vi "Update Display Message.vi"(8 "error in (no error)":errorcluster, 10 "Wash Steps Selected-Update Display Message In":T1, 11 "Data Cluster":T2) -> (0 "error out":errorcluster, 1 "Step in progress timer control":variant, 2 "Wash Steps Selected-Update Display Message Out":T1)   [LabVIEW 2020]
doc: "Updates the Front Panel."
uses:
  Controls/Car Wash References.ctl
  Controls/Wash Steps Selected-Update Display Message.ctl
  Controls/Timer Controls.ctl
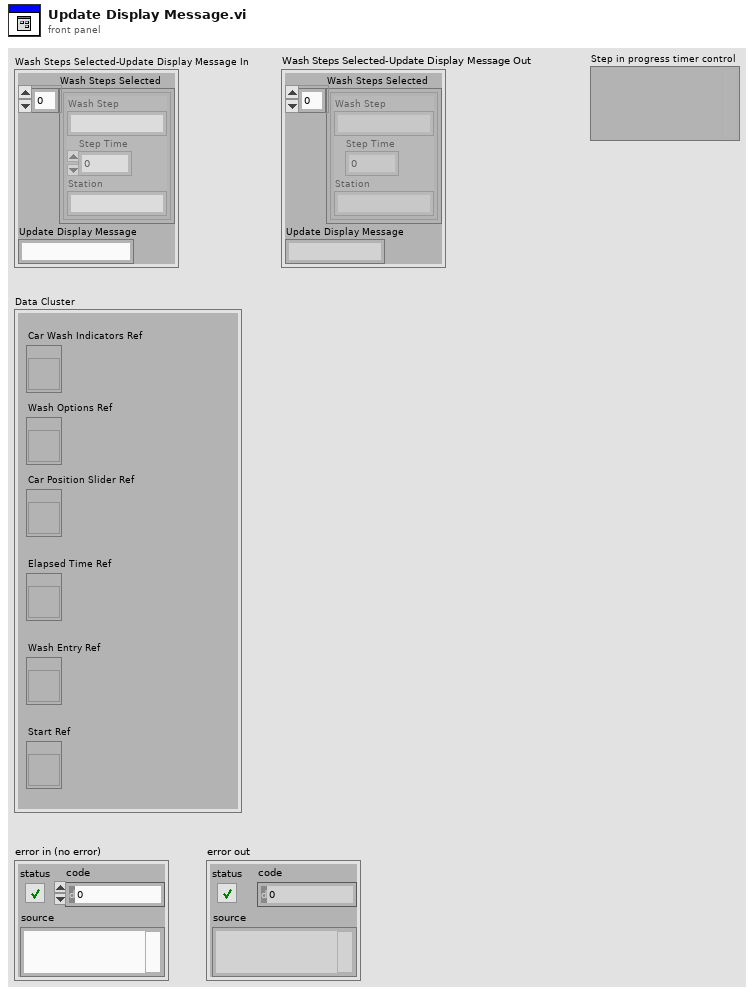
[diagram p1: front panel]
types:
  T1 = typedef "Wash Steps Selected-Update Display Message.ctl" = cluster{"Wash Steps Selected":cluster{"Wash Step":string, "Step Time":i32, "Station":string}[], "Update Display Message":string}
  T2 = typedef "Car Wash References.ctl" = cluster{"Car Wash Indicators Ref":refnum<vi>, "Wash Options Ref":refnum<vi>, "Car Position Slider Ref":refnum<vi>, "Elapsed Time Ref":refnum<vi>, "Wash Entry Ref":refnum<vi>, "Start Ref":refnum<vi>}
  T3 = enum8{"Enabled", "Disabled", "Disabled and Grayed Out"}
  T4 = cluster{"Wash Step":string, "Step Time":i32, "Station":string}[]
  T5 = typedef "Timer Controls.ctl" = enum16{"Reset", "Start", "Stop"}
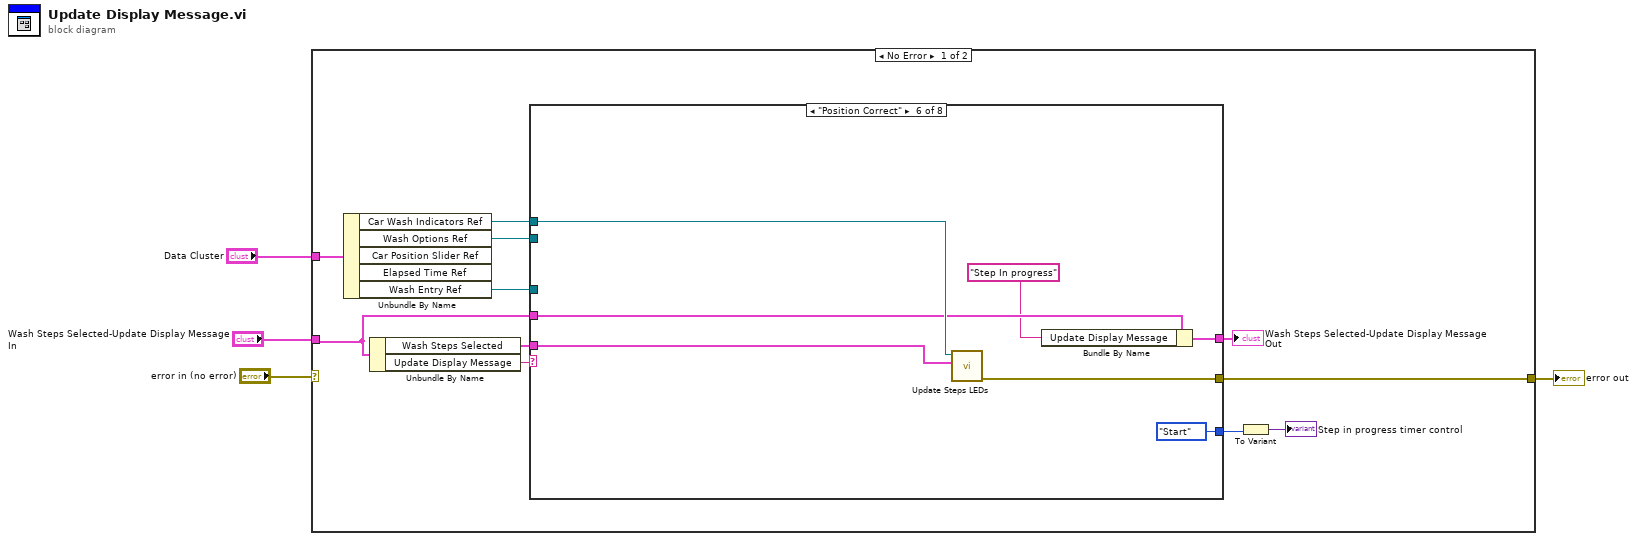
[diagram p0: block diagram]
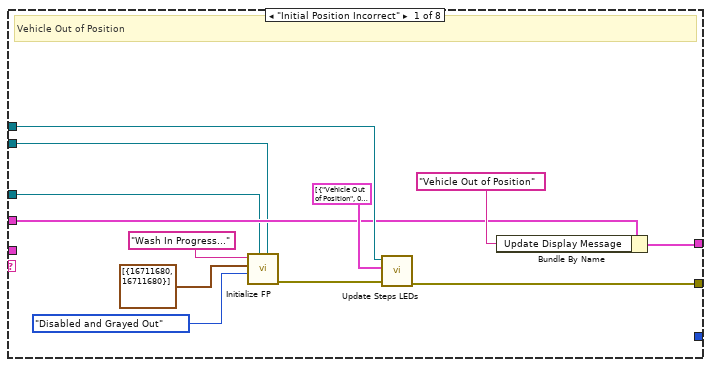
[diagram p2: hidden frame]
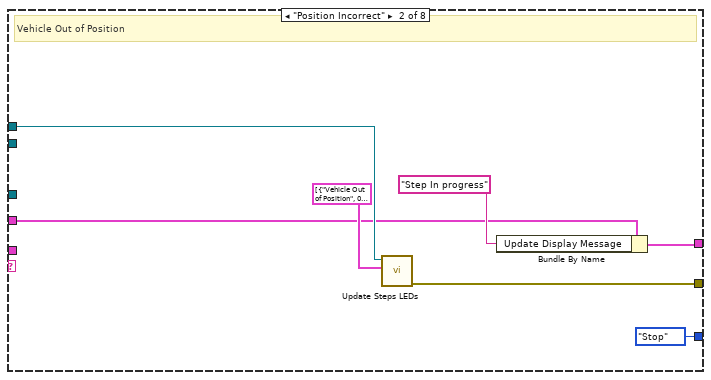
[diagram p3: hidden frame]
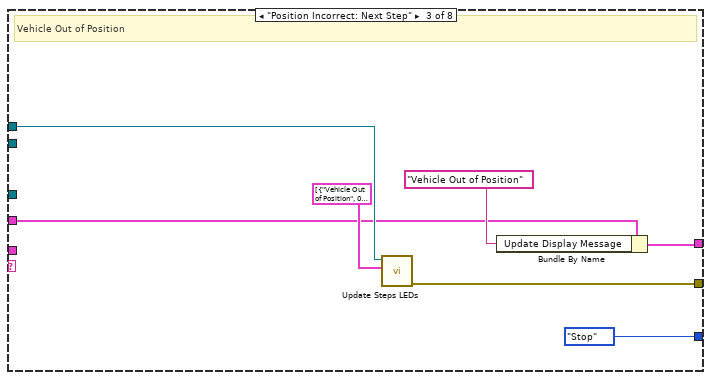
[diagram p4: hidden frame]
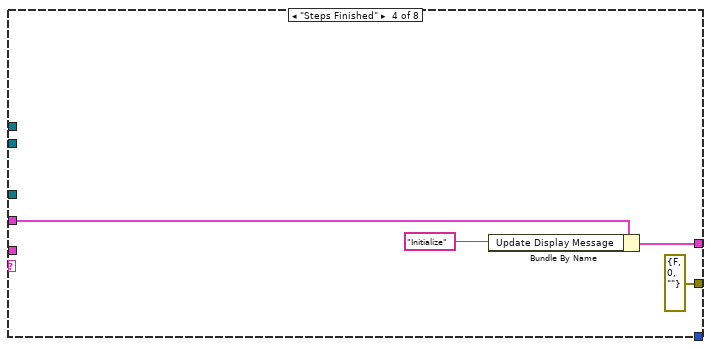
[diagram p5: hidden frame]
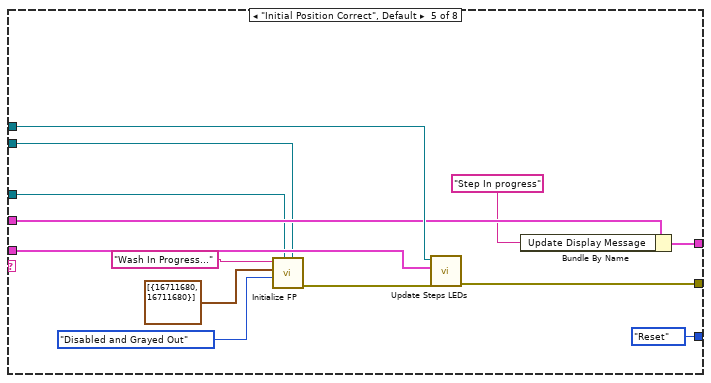
[diagram p6: hidden frame]
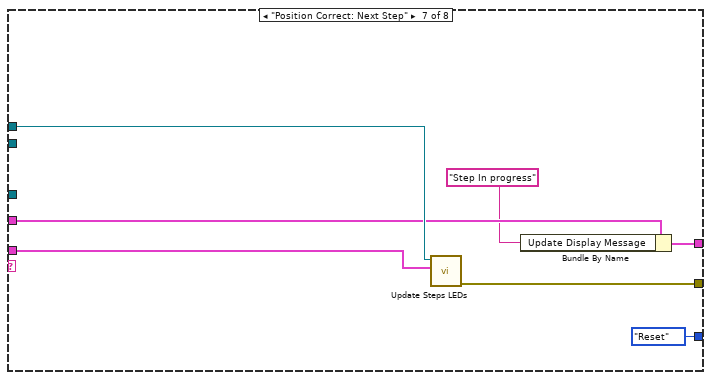
[diagram p7: hidden frame]
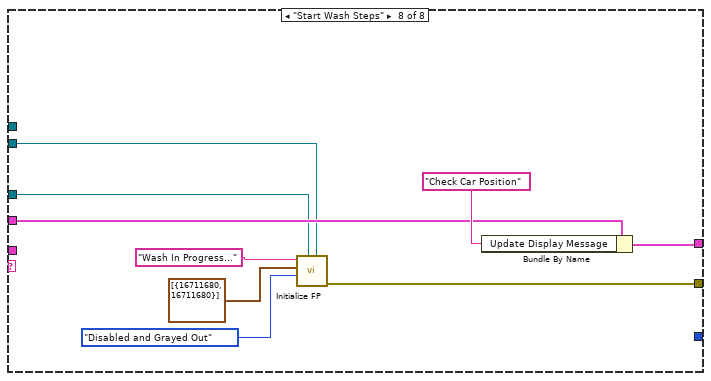
[diagram p8: hidden frame]
diagram:
  n1 = case shown="No Error" "error in (no error)" {
    selector: "error in (no error)" -> [_ w82]
    tunnel: "Data Cluster" -> [w14 _]
    tunnel: [w10 w82] -> w2
    tunnel: "Wash Steps Selected-Update Display Message In" -> [w8 _]
    frame No Error {
      n2 = Unbundle By Name(w14) -> ("Car Wash Indicators Ref"=w12:refnum<vi>, "Wash Options Ref"=w7:refnum<vi>, "Wash Entry Ref"=w13:refnum<vi>)  [unwired: 2 out]
      n3 = Unbundle By Name(w8) -> ("Wash Steps Selected"=w11:T4, "Update Display Message"=w15:string)
      n4 = case shown="\"Position Correct\"" w15 {
        tunnel: w13 -> [w18 _ _ _ w47 _ _ w74]
        tunnel: w12 -> [w25 w32 w39 _ w58 w65 w72 _]
        tunnel: w11 -> [_ _ _ _ w57 w64 w71 _]
        tunnel: [w26 w33 w40 errorcluster {"status"=FALSE, "code"=0, "source"=""} ("error out") w56 w63 w70 w75] -> w10
        tunnel: w8 -> [w23 w30 w37 w44 w55 w62 w69 w79]
        tunnel: [w22 w29 w36 w43 w54 w61 w68 w80] -> w9
        tunnel: w7 -> [w17 _ _ _ w46 _ _ w73]
        tunnel: [_ Timer_Controls."Stop" ("Enum") Timer_Controls."Stop" ("Enum") _ Timer_Controls."Reset" ("Enum") Timer_Controls."Start" ("Enum") Timer_Controls."Reset" ("Enum") _] -> w5
        frame "Initial Position Incorrect" {
          # "Vehicle Out of Position"
          n5 = call "Initialize FP.vi"("Wash Options Ref"=w17, "Wash Entry Ref"=w18, "Enable\\Disable Wash Options"=T3."Disabled and Grayed Out" ("Enable\\Disable Wash Options"), "Wash In Progress Color"=cluster{u32, u32}[] [{16711680, 16711680}], "Wash In Progress Text"="Wash In Progress...") -> ("error out"=w16:errorcluster)  [unwired: 6 in]
          n6 = call "Update Steps LEDs.vi"("error in"=w16, "Wash Steps Selected"=T4 [{"Wash Step"="Vehicle Out of Position", "Step Time"=0, "Station"=""}], "Car Wash Indicators Ref"=w25) -> ("error out"=w26:errorcluster)  [unwired: 8 in]
          n7 = Bundle By Name(cluster=w23, "Update Display Message"="Vehicle Out of Position") -> (w22:T1)
        }
        frame "Position Incorrect" {
          # "Vehicle Out of Position"
          n8 = call "Update Steps LEDs.vi"("Wash Steps Selected"=T4 [{"Wash Step"="Vehicle Out of Position", "Step Time"=0, "Station"=""}], "Car Wash Indicators Ref"=w32) -> ("error out"=w33:errorcluster)  [unwired: 9 in]
          n9 = Bundle By Name(cluster=w30, "Update Display Message"="Step In progress") -> (w29:T1)
        }
        frame "Position Incorrect: Next Step" {
          # "Vehicle Out of Position"
          n10 = call "Update Steps LEDs.vi"("Wash Steps Selected"=T4 [{"Wash Step"="Vehicle Out of Position", "Step Time"=0, "Station"=""}], "Car Wash Indicators Ref"=w39) -> ("error out"=w40:errorcluster)  [unwired: 9 in]
          n11 = Bundle By Name(cluster=w37, "Update Display Message"="Vehicle Out of Position") -> (w36:T1)
        }
        frame "Steps Finished" {
          n12 = Bundle By Name(cluster=w44, "Update Display Message"="Initialize") -> (w43:T1)
        }
        frame "Initial Position Correct", Default {
          n13 = call "Initialize FP.vi"("Wash Options Ref"=w46, "Wash Entry Ref"=w47, "Enable\\Disable Wash Options"=T3."Disabled and Grayed Out" ("Enable\\Disable Wash Options"), "Wash In Progress Color"=cluster{u32, u32}[] [{16711680, 16711680}], "Wash In Progress Text"="Wash In Progress...") -> ("error out"=w48:errorcluster)  [unwired: 6 in]
          n14 = call "Update Steps LEDs.vi"("error in"=w48, "Wash Steps Selected"=w57, "Car Wash Indicators Ref"=w58) -> ("error out"=w56:errorcluster)  [unwired: 8 in]
          n15 = Bundle By Name(cluster=w55, "Update Display Message"="Step In progress") -> (w54:T1)
        }
        frame "Position Correct" {
          n16 = call "Update Steps LEDs.vi"("Wash Steps Selected"=w64, "Car Wash Indicators Ref"=w65) -> ("error out"=w63:errorcluster)  [unwired: 9 in]
          n17 = Bundle By Name(cluster=w62, "Update Display Message"="Step In progress") -> (w61:T1)
        }
        frame "Position Correct: Next Step" {
          n18 = call "Update Steps LEDs.vi"("Wash Steps Selected"=w71, "Car Wash Indicators Ref"=w72) -> ("error out"=w70:errorcluster)  [unwired: 9 in]
          n19 = Bundle By Name(cluster=w69, "Update Display Message"="Step In progress") -> (w68:T1)
        }
        frame "Start Wash Steps" {
          n20 = call "Initialize FP.vi"("Wash Options Ref"=w73, "Wash Entry Ref"=w74, "Enable\\Disable Wash Options"=T3."Disabled and Grayed Out" ("Enable\\Disable Wash Options"), "Wash In Progress Color"=cluster{u32, u32}[] [{16711680, 16711680}], "Wash In Progress Text"="Wash In Progress...") -> ("error out"=w75:errorcluster)  [unwired: 6 in]
          n21 = Bundle By Name(cluster=w79, "Update Display Message"="Check Car Position") -> (w80:T1)
        }
      }
      "Wash Steps Selected-Update Display Message Out" <- w9
      n22 = To Variant(anything=w5) -> (Variant=→"Step in progress timer control":variant)
    }
    frame Error {
    }
  }
  "error out" <- w2
